vi "Convert Database Value To Class.vi"(8 "error in (no error)":errorcluster, 9 "SQL query":string, 10 "Table":string="Select * from xx", 11 "MemberInfo in":refnum<class "Information.lvclass">) -> (0 "error out":errorcluster, 3 "MemberInfo out":refnum<class "Information.lvclass">)   [LabVIEW 2015, in "Information.lvclass"]
uses:
  Information.lvclass
  <vilib>/addons/database/Auxilliary.llb/DB Tools Column Info.ctl
  <vilib>/addons/database/Auxilliary.llb/DB Tools DataTypes.ctl
  Information.lvclass/Information.ctl
  API/_Database/Database.lvclass
  <vilib>/addons/database/NI_Database_API.lvlib
  Type Definitions/Main Ctl and VI ref.ctl
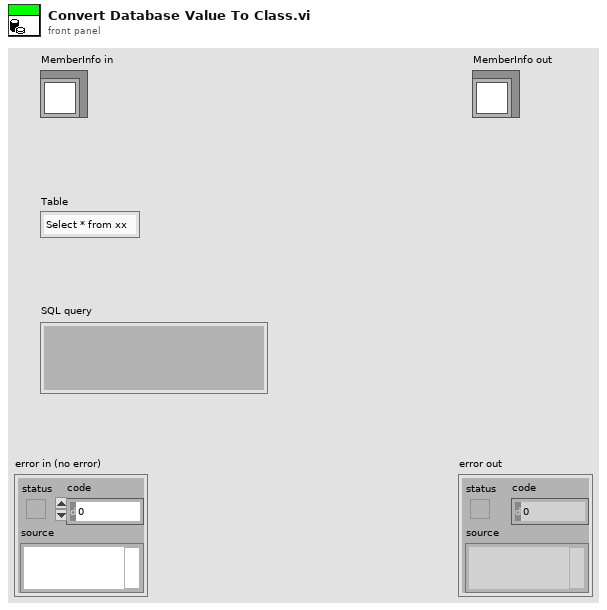
[diagram p1: front panel]
types:
  T1 = typedef "NI_Database_API.lvlib/DB Tools Column Info.ctl" = cluster{"column name":string, "data type":T2, "size":i32, "allow null?":bool}
  T2 = typedef "NI_Database_API.lvlib/DB Tools DataTypes.ctl" = enum16{"String", "Long (I32)", "Single (SGL)", "Double (DBL)", "Date/Time", "Binary"}
  T3 = typedef "Information.lvclass/Main Ctl and VI ref.ctl" = cluster{"姓名":refnum<vi>, "年级":refnum<vi>, "学号":refnum<vi>, "照片":refnum<vi>, "性别":refnum<vi>, "邮箱":refnum<vi>, "电话":refnum<vi>, "QQ":refnum<vi>, "学院":refnum<vi>, "点击上传照片":refnum<vi>, "操作资料":refnum<vi>, "部门":refnum<vi>, "组别":refnum<vi>, "UI_Enable":refnum<vi>}
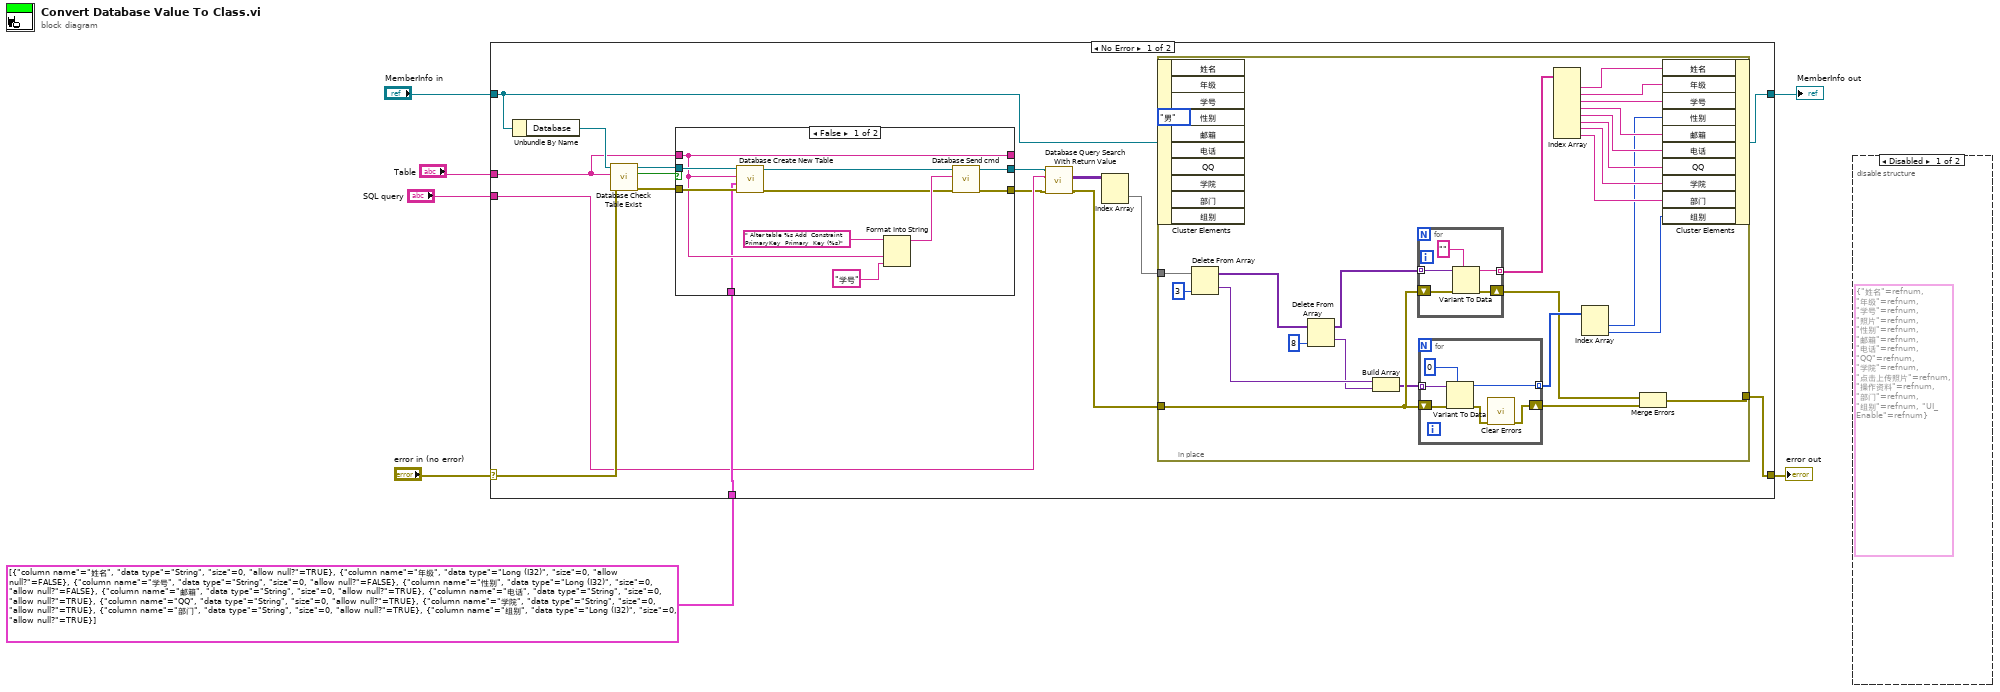
[diagram p0: block diagram]
diagram:
  n1 = case shown="No Error" "error in (no error)" {
    selector: "error in (no error)" -> [w22 w74]
    tunnel: [w9 w74] -> w6
    tunnel: [w8 w73] -> w4
    tunnel: "MemberInfo in" -> [w12 w73]
    tunnel: "SQL query" -> [w15 _]
    tunnel: "Table" -> [w18 _]
    tunnel: T1[] [{"column name"="姓名", "data type"=enum."String", "size"=0, "allow null?"=TRUE}, {"column name"="年级", "data type"=enum."Long (I32)", "size"=0, "allow null?"=FALSE}, {"column name"="学号", "data type"=enum."String", "size"=0, "allow null?"=FALSE}, {"column name"="性别", "data type"=enum."Long (I32)", "size"=0, "allow null?"=FALSE}, {"column name"="邮箱", "data type"=enum."String", "size"=0, "allow null?"=TRUE}, {"column name"="电话", "data type"=enum."String", "size"=0, "allow null?"=TRUE}, {"column name"="QQ", "data type"=enum."String", "size"=0, "allow null?"=TRUE}, {"column name"="学院", "data type"=enum."String", "size"=0, "allow null?"=TRUE}, {"column name"="部门", "data type"=enum."String", "size"=0, "allow null?"=TRUE}, {"column name"="组别", "data type"=enum."Long (I32)", "size"=0, "allow null?"=TRUE}] ("column information") -> [w17 _]
    frame No Error {
      n2 = Unbundle By Name(w12) -> ("Database"=w23:refnum<class "Database.lvclass">)
      n3 = call "Database Check Table Exist.vi"("error in (no error)"=w22, "Table"=w18, "Database in"=w23) -> ("error out"=w21:errorcluster, "Exit?"=w20:bool, "Database out"=w19:refnum<class "Database.lvclass">)  [unwired: 6 in]
      n4 = case shown="False" w20 {
        tunnel: w19 -> [w69 w71]
        tunnel: w21 -> [w68 w72]
        tunnel: w18 -> [w60 w70]
        tunnel: [w62 w72] -> w14
        tunnel: [w61 w71] -> w16
        tunnel: [w60 w70] -> _
        tunnel: w17 -> [w59 _]
        frame False {
          n5 = call "Database Create New Table.vi"("error in (no error)"=w68, "column information"=w59, "table"=w60, "Database in"=w69) -> ("error out"=w64:errorcluster, "Database out"=w63:refnum<class "Database.lvclass">)  [unwired: 6 in]
          n6 = Format Into String(format string=" Alter table %s Add  Constraint  PrimaryKey  Primary  Key (%s)" ("SQL query"), w60, "学号" ("input 2")) -> (resulting string=w67:string)  [unwired: 2 in, 1 out]
          n7 = call "Database Send cmd.vi"("error in (no error)"=w64, "SQL query"=w67, "Database in"=w63) -> ("error out"=w62:errorcluster, "Database out"=w61:refnum<class "Database.lvclass">)  [unwired: 7 in]
        }
        frame True {
        }
      }
      n8 = call "Database Query Search With Return Value.vi"("error in (no error)"=w14, "SQL query"=w15, "object in"=w16) -> ("error out"=w10:errorcluster, "recordset data"=w13:variant[][])  [unwired: 5 in, 2 out]
      n9 = Index Array(array=w13) -> (element=w11:variant[])  [unwired: 2 in]
      n10 = in-place {
        in-place-border: w11 -> [w47]
        in-place-border: w10 -> [w41]
        in-place-border: [w30] -> w9
        (unwired) enum16{"男", "女"}."男" ("UserInfo.性别")
        n11 = in-place-cluster #1(w12) -> ()  [unwired: 10 out]
        n12 = Delete From Array(array=w47, index=3) -> (deleted portion=w43:variant, array with subset deleted=w45:variant[])  [unwired: 1 in]
        n13 = Delete From Array(array=w45, index=8) -> (deleted portion=w42:variant, array with subset deleted=w28:variant[])  [unwired: 1 in]
        n14 = Build Array(w43, w42) -> (w29:variant[])
        n15 = for {
          tunnel: w28 -> [w58] mode=indexing
          tunnel: [w56] -> w40 mode=indexing
          shift-right: [w54] -> w31
          shift-left: w41 -> [w55]
          n16 = Variant To Data(error in=w55, type="", Variant=w58) -> (data=w56:string, error out=w54:errorcluster)
        }
        n17 = for {
          tunnel: w29 -> [w53] mode=indexing
          tunnel: [w50] -> w33 mode=indexing
          shift-right: [w48] -> w32
          shift-left: w41 -> [w51]
          n18 = Variant To Data(error in=w51, type=0, Variant=w53) -> (data=w50:i32, error out=w49:errorcluster)
          n19 = call <vilib>:"Clear Errors.vi"("error in (no error)"=w49) -> ("error out"=w48:errorcluster)  [unwired: 5 in, 1 out]
        }
        n20 = Index Array(array=w40) -> (element #1=w25:string, element #2=w24:string, element #3=w39:string, element #4=w38:string, element #5=w37:string, element #6=w36:string, element #7=w35:string, element #8=w34:string)  [unwired: 8 in]
        n21 = Index Array(array=w33) -> (element #1=w27:i32, element #2=w26:i32)  [unwired: 2 in]
        n22 = Merge Errors(w31, w32) -> (w30:errorcluster)
        n23 = in-place-cluster #1("姓名"=w25, "年级"=w24, "学号"=w39, "性别"=w27, "邮箱"=w38, "电话"=w37, "QQ"=w36, "学院"=w35, "部门"=w34, "组别"=w26) -> (w8:refnum<class "Information.lvclass">)
      }
    }
    frame Error {
    }
  }
  "error out" <- w6
  "MemberInfo out" <- w4
  n24 = disable-structure shown="Disabled" {
    frame Disabled {
      (unwired) T3 {"姓名"=refnum, "年级"=refnum, "学号"=refnum, "照片"=refnum, "性别"=refnum, "邮箱"=refnum, "电话"=refnum, "QQ"=refnum, "学院"=refnum, "点击上传照片"=refnum, "操作资料"=refnum, "部门"=refnum, "组别"=refnum, "UI_Enable"=refnum} ("Refs")
    }
    frame Enabled {
    }
  }
